vi "5_Manual Window.vi"() -> ()   [LabVIEW 2015]
uses:
  PLC Commucation/Motor cmd setting.ctl
  PLC Commucation/Motor Action.ctl
  PLC Commucation/Motor Selection.ctl
  Variable/Default Setting.ctl
  Variable/Global.vi
  <vilib>/Utility/file.llb/Write To Spreadsheet File (DBL).vi
  <vilib>/Utility/file.llb/Read From Spreadsheet File (DBL).vi
panel:
  in  "Y-Axis-Home":bool
  out "Default Setting":T1
  out "Voltage":dbl
  out "PLC Send CMD":string="*IDN?\n"
  in  "DIGITAL OUTPUT":T2
  in  "Free Axis  RUN":bool
  in  "Free Axis Lock":bool
  in  "Speed(RPM)":i16(knob) max=5000 scale=0.0..5000.0
  in  "X-Axis Save":bool
  in  "Y-Axis Save":bool
  in  "Z-Axis Save":bool
  in  "Z-Axis-Home":bool
  in  "X-Axis-Home":bool
  out "DIGITAL INPUT":T3
  out "Z Actual Position":dbl caption="Actual Position"
  out "Y Actual Position":dbl caption="Actual Position"
  out "X Actual Position":dbl caption="Actual Position"
  in  "Z Axis Run":bool
  in  "Y Axis Run":bool
  in  "X Axis Run":bool
  in  "Z Axis Lock":bool
  in  "X Axis Lock":bool
  in  "Y Axis Lock":bool
  in  "Z-Axis Speed":i16(knob) max=50 scale=0.0..50.0
  in  "Y-Axis Speed":i16(knob) max=50 scale=0.0..50.0
  in  "X-Axis Speed":i16(knob) max=50 scale=0.0..50.0
  out "Receieve CMD":string
  in  "Motor Setting":T4
  out "exit":bool
  in  "Status":bool[](array[boolean])
  in  "zero":bool
  in  "back":bool
  in  "save":bool
  # "Manual Mode Screen"
  # "FREE-Axis"
  # "X-Axis"
  # "Y-Axis"
  # "Z-Axis"
  # "Developed by: VR Engineers"
  # "Contact: 9891971134"
  # "DIGITAL OUTPUT"
  # "DIGITAL OUTPUT"
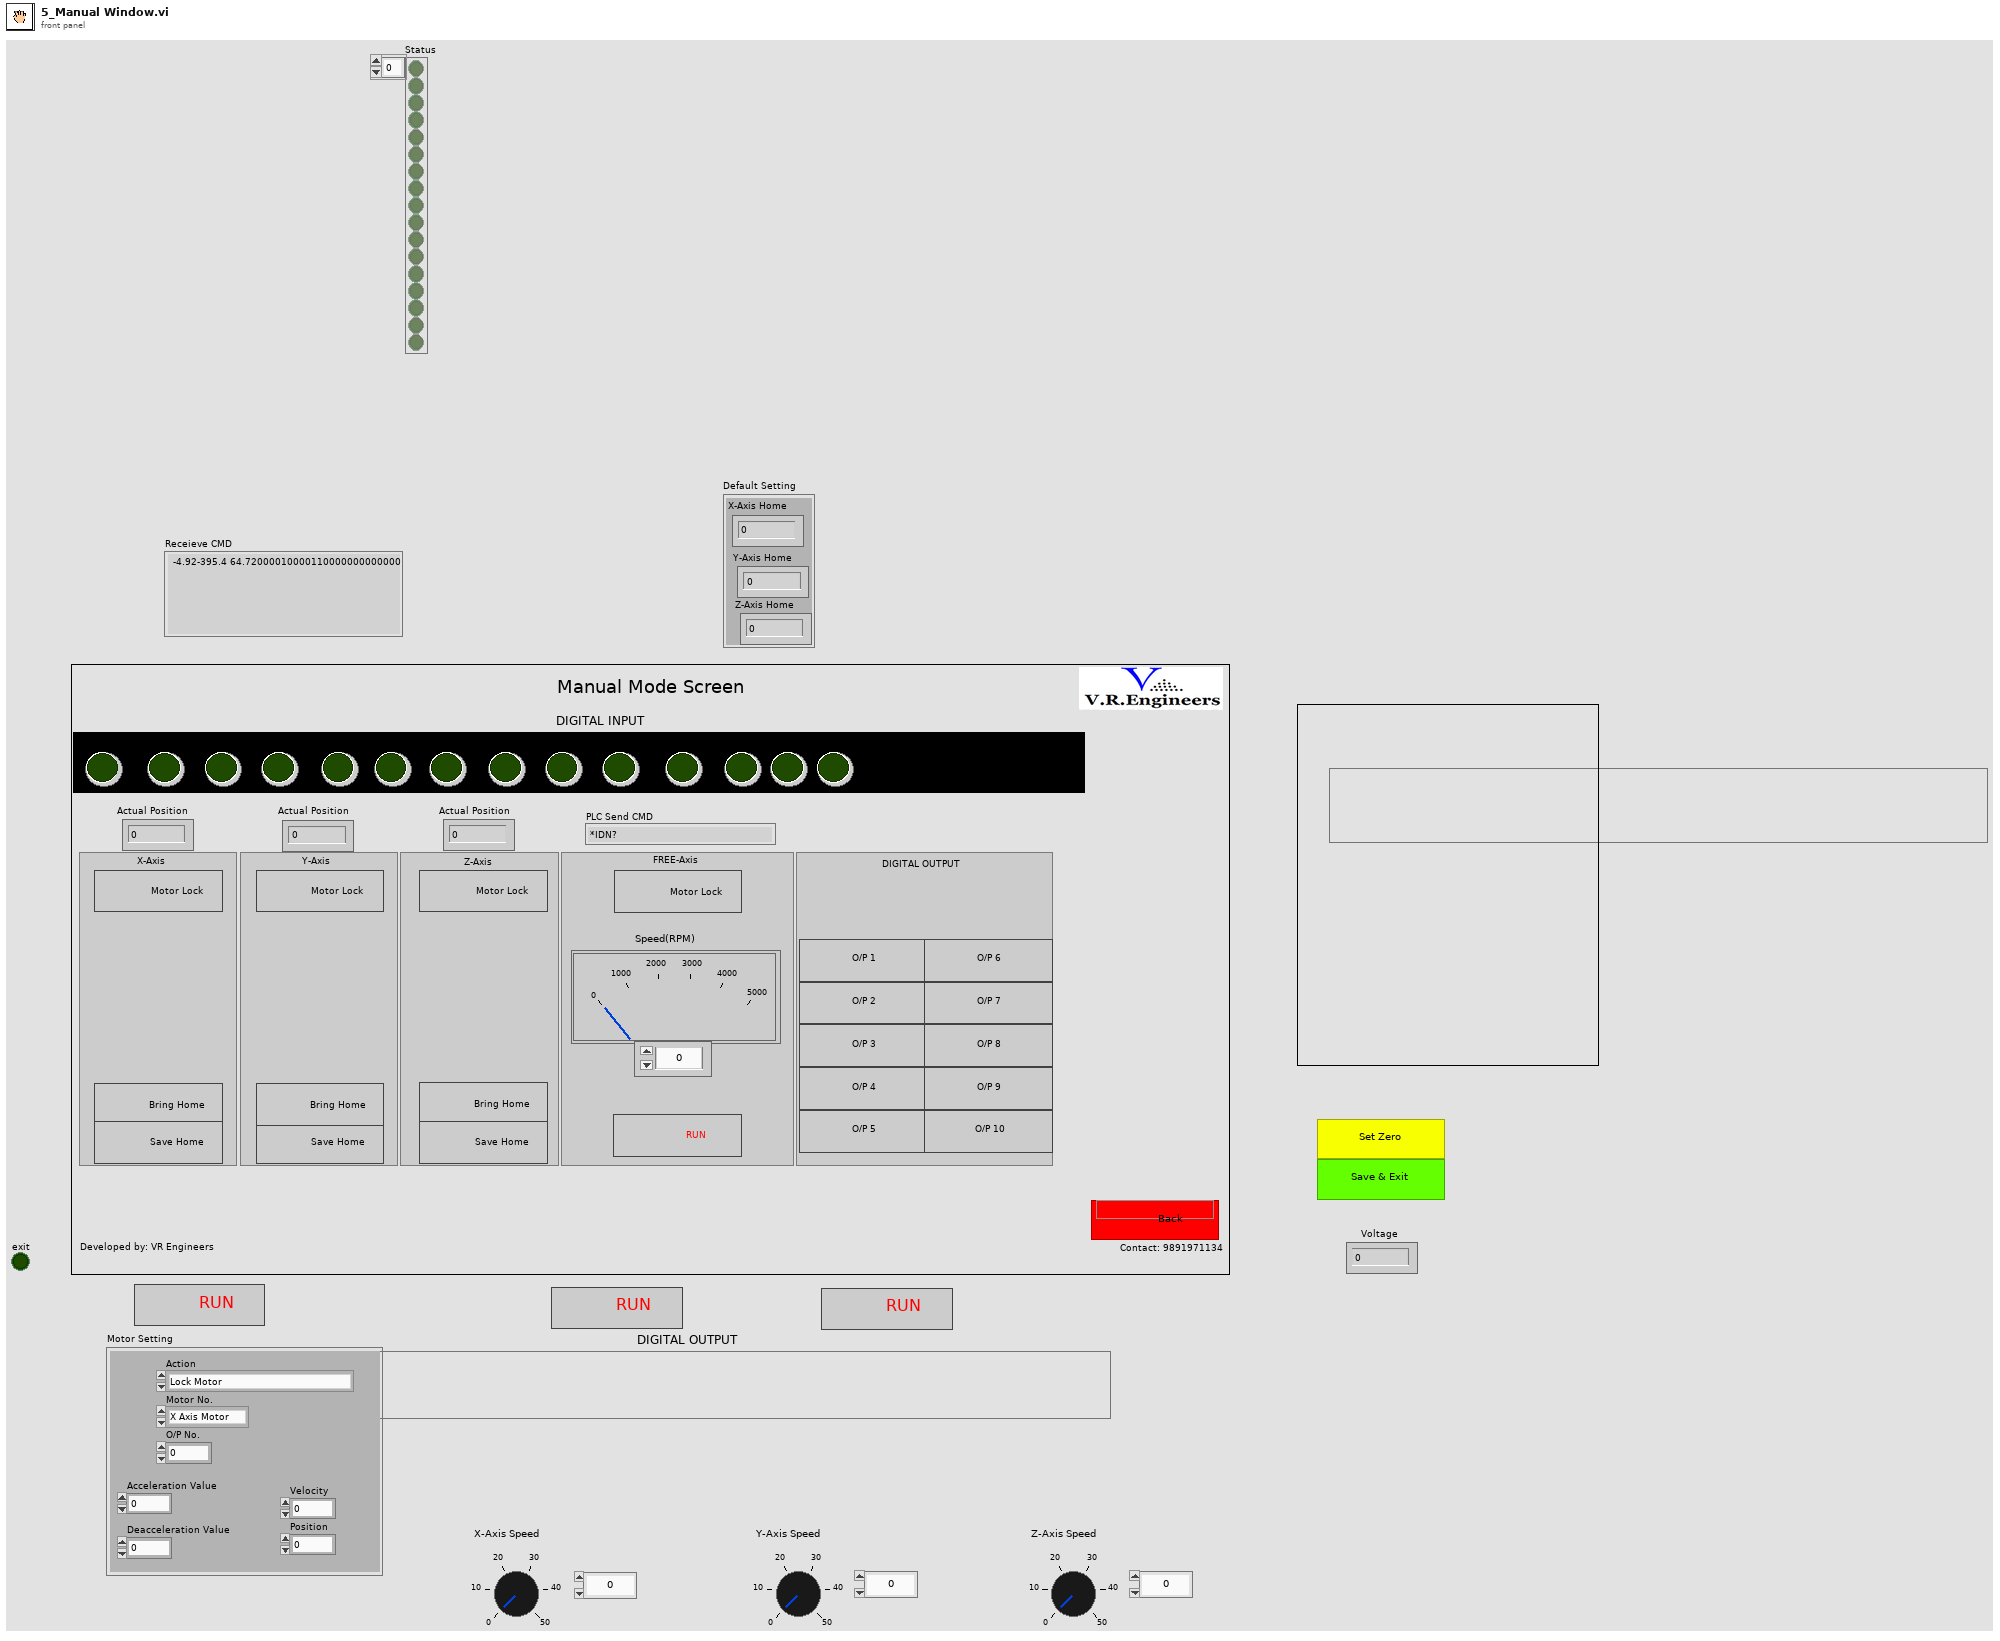
[diagram p1: front panel]
types:
  T1 = typedef "Default Setting.ctl" = cluster{"X-Axis Home":dbl, "Y-Axis Home":dbl, "Z-Axis Home":dbl}
  T2 = cluster{"0":bool, "1":bool, "2":bool, "3":bool, "4":bool, "5":bool, "6":bool, "7":bool, "8":bool, "9":bool}
  T3 = cluster{"Y Axis FWD":bool, "Z Axis DOWN":bool, "Z Axis UP":bool, "X Axis RIGHT":bool, "Y Axis REV":bool, "X Axis LEFT":bool, "X Axis Start":bool, "Y Axis Start":bool, "Z Axis Start":bool, "Emergency":bool, "JOG FWD/REV":bool, "SPI_0011":bool, "SPI_0012":bool, "SPI_0013":bool}
  T4 = typedef "Motor cmd setting.ctl" = cluster{"Action":T5, "Motor No.":T6, "O/P No.":i16, "Acceleration Value":dbl, "Deacceleration Value":dbl, "Position":dbl, "Velocity":dbl}
  T5 = typedef "Motor Action.ctl" = enum16{"Lock Motor", "Unlock Motor", "Set Position Value", "Set Velocity", "Set Acceleration", "Set Deceleration", "Start Motor", "Stop Motor", "Set Home Position", "ALL Servo Home", "Output ON", "Outout OFF"}
  T6 = typedef "Motor Selection.ctl" = enum16{"X Axis Motor", "Y Axis Motor", "Z Axis Motor", "Free Axis Motor"}
  T7 = enum16{"open", "replace", "create", "open or create", "replace or create", "replace or create with confirmation"}
  T8 = enum16{"big-endian, network order", "native, host order", "little-endian"}
  T9 = cluster{"DI[0]":bool, "DI[1]":bool, "DI[2]":bool, "DI[3]":bool, "DI[4]":bool, "DI[5]":bool, "DI[6]":bool, "DI[7]":bool, "DI[8]":bool, "DI[9]":bool, "DI[10]":bool, "DI[11]":bool, "DI[12]":bool, "DI[13]":bool}
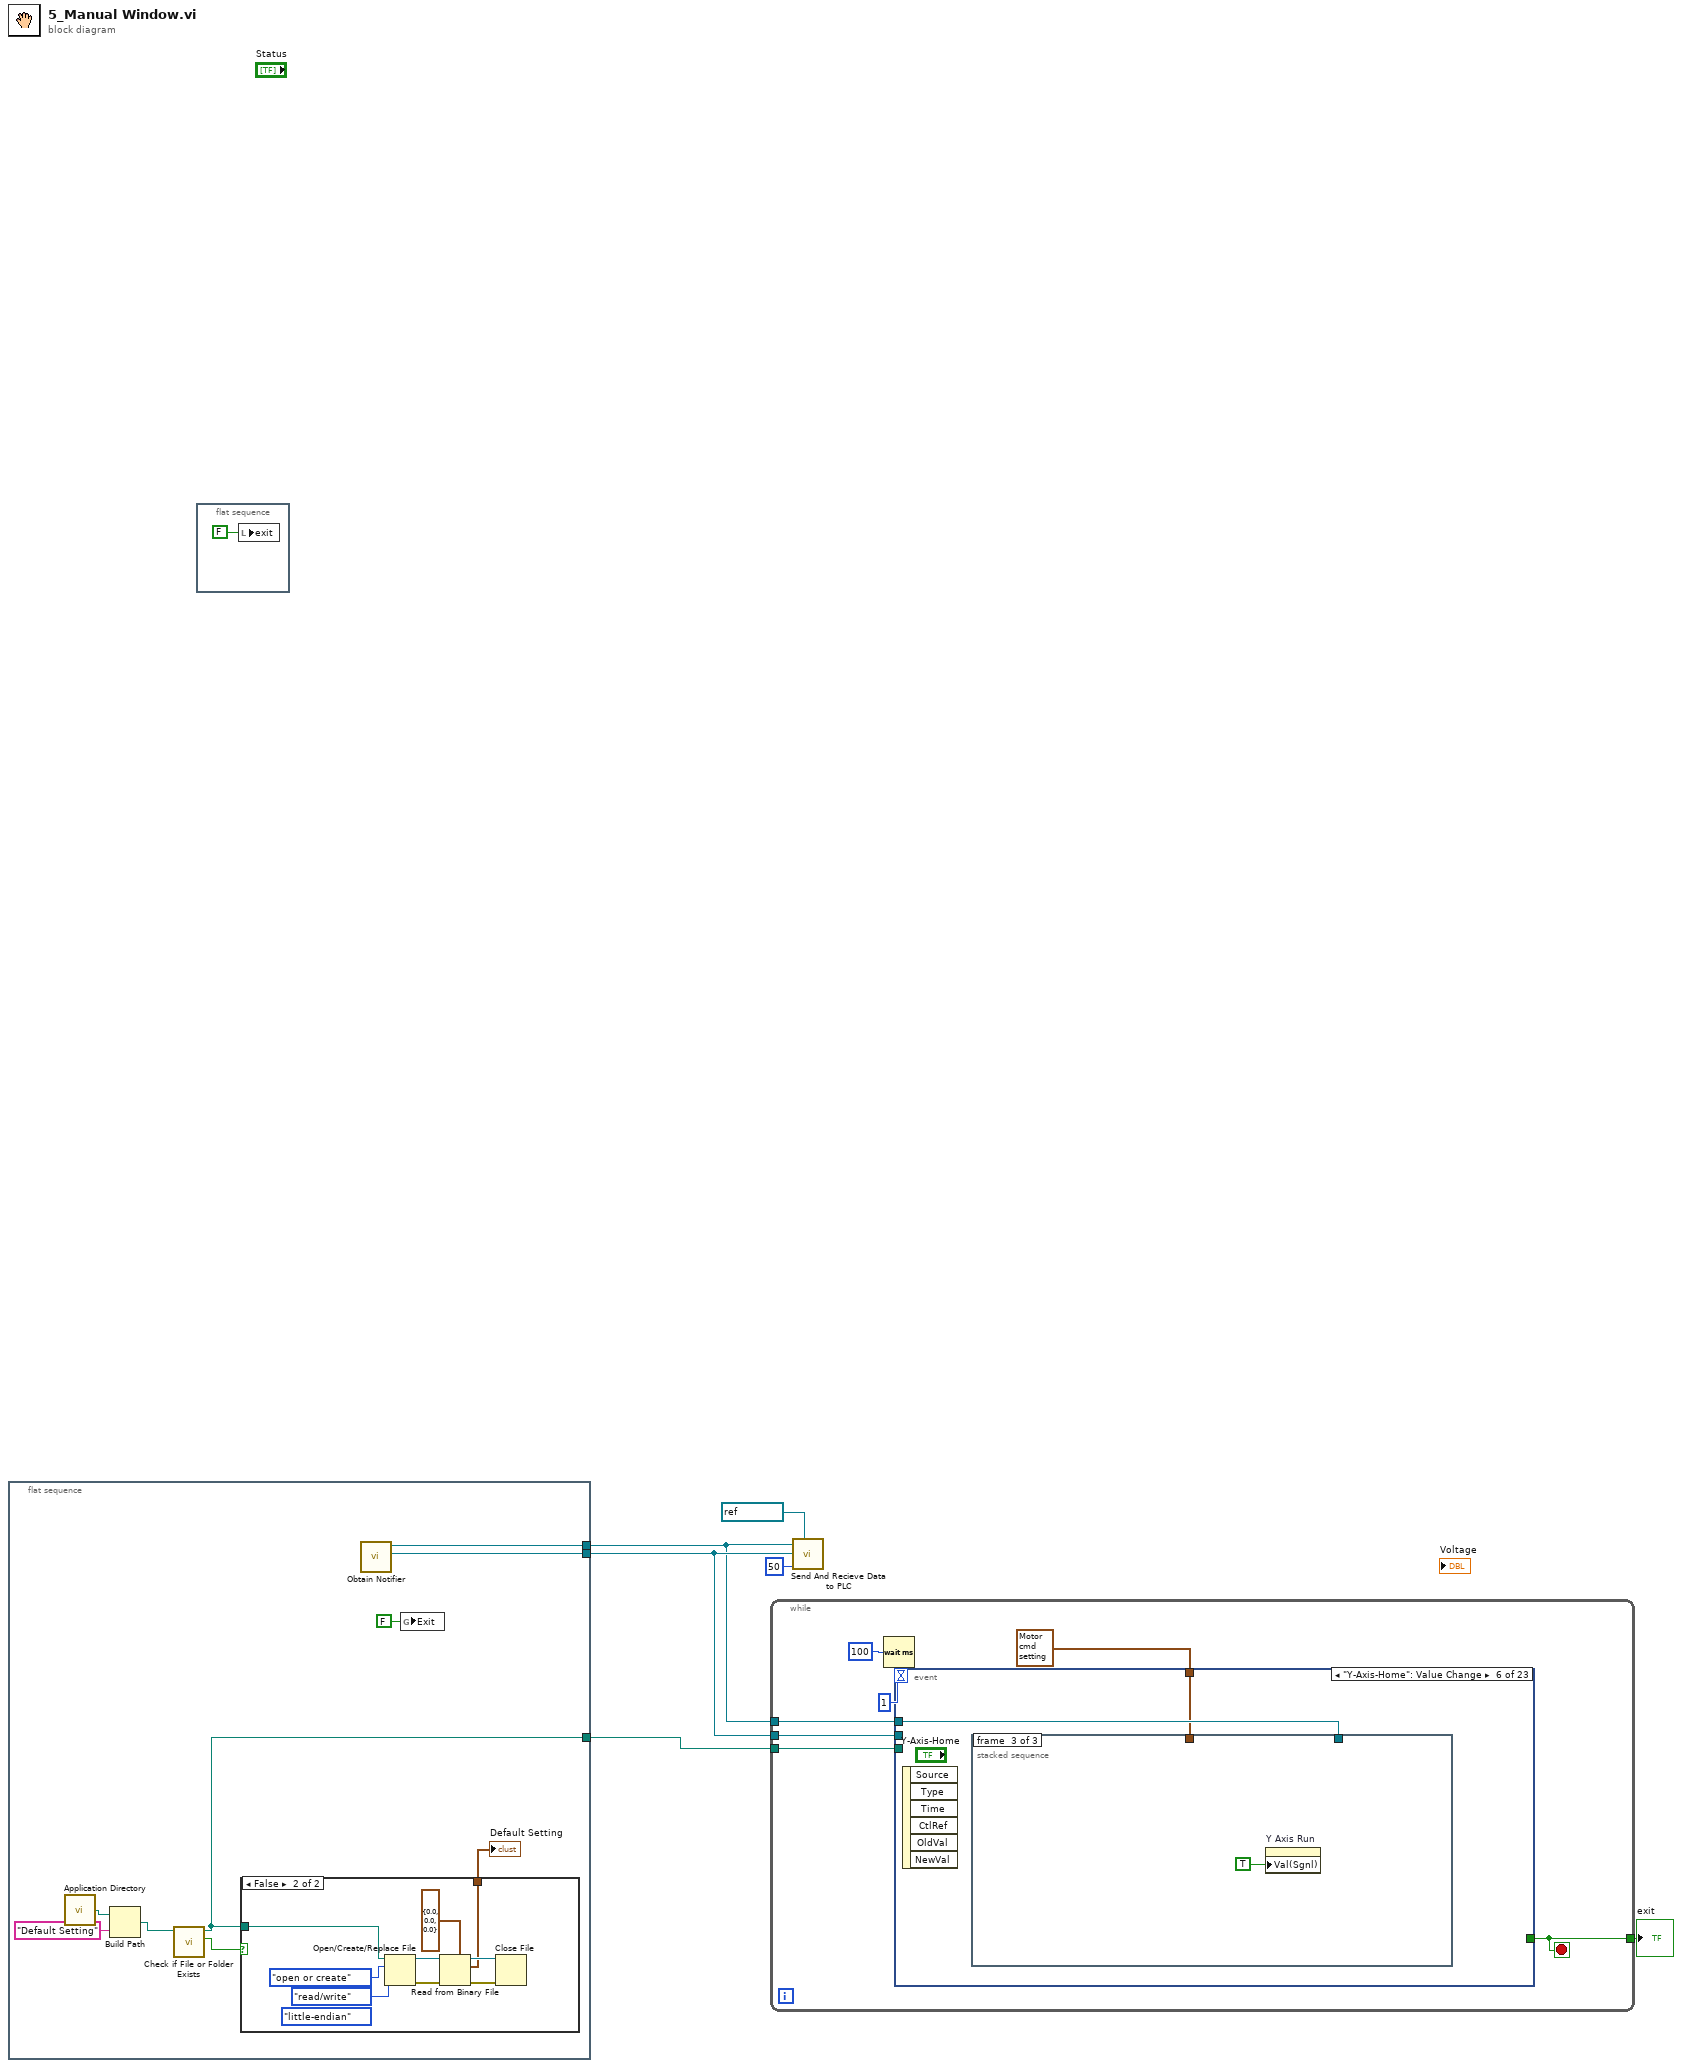
[diagram p0: block diagram]
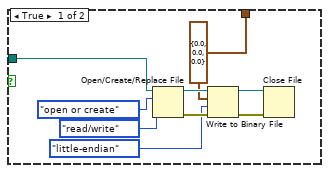
[diagram p2: hidden frame]
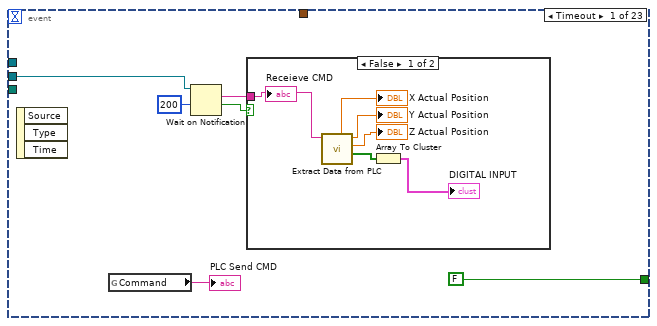
[diagram p3: hidden frame]
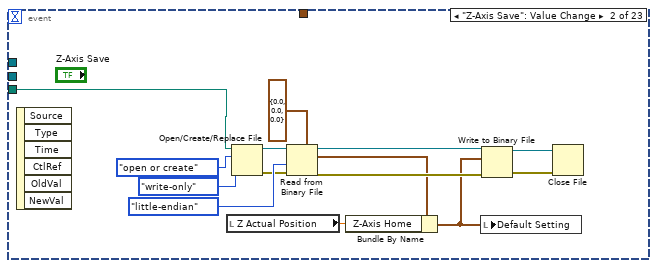
[diagram p5: hidden frame]
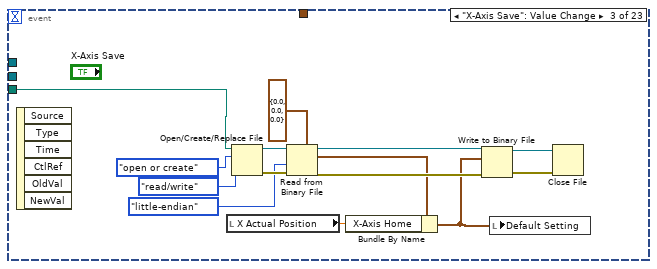
[diagram p6: hidden frame]
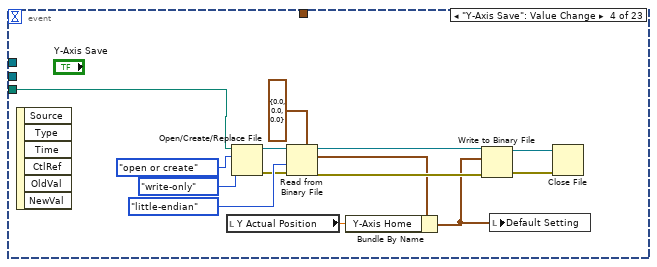
[diagram p7: hidden frame]
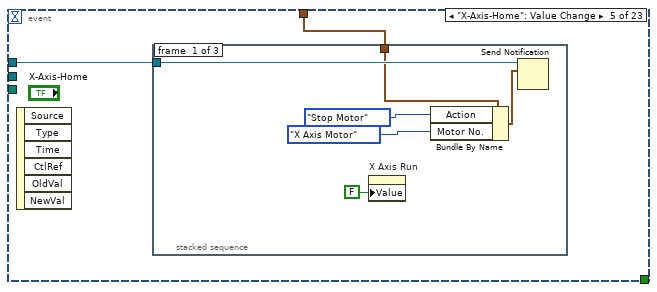
[diagram p8: hidden frame]
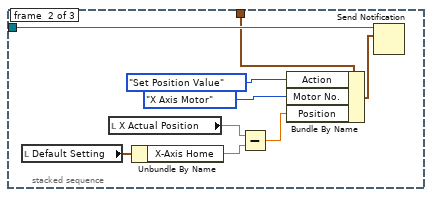
[diagram p9: hidden frame]
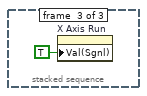
[diagram p10: hidden frame]
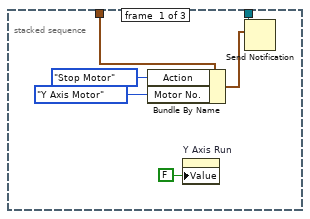
[diagram p11: hidden frame]
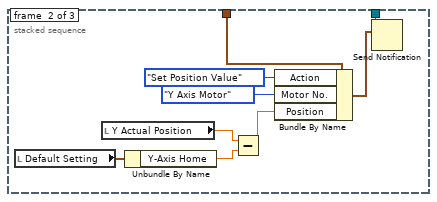
[diagram p12: hidden frame]
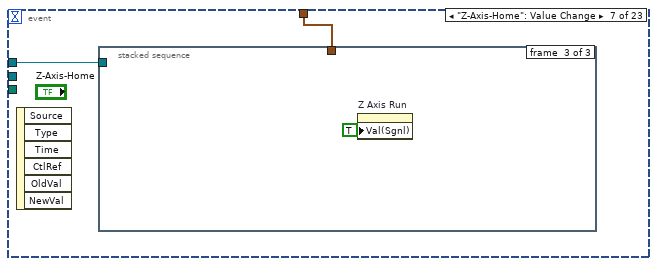
[diagram p13: hidden frame]
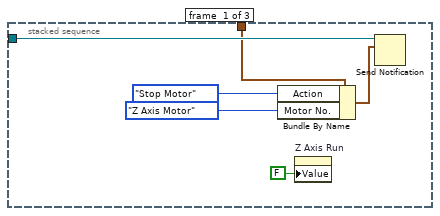
[diagram p14: hidden frame]
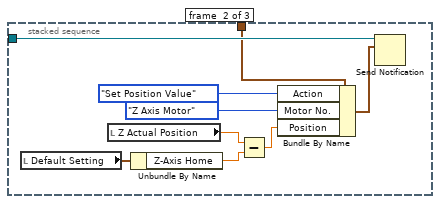
[diagram p15: hidden frame]
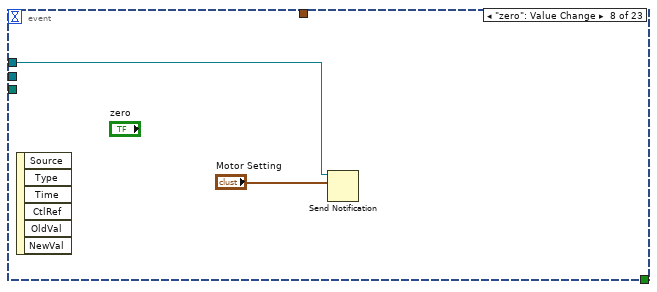
[diagram p16: hidden frame]
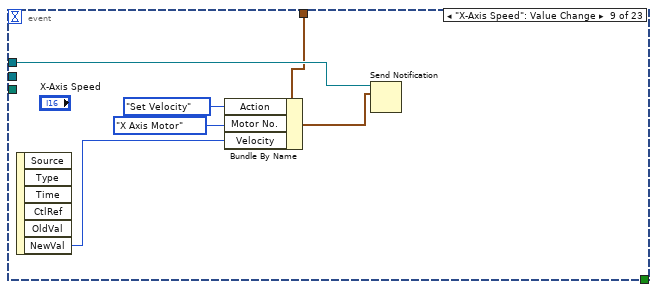
[diagram p17: hidden frame]
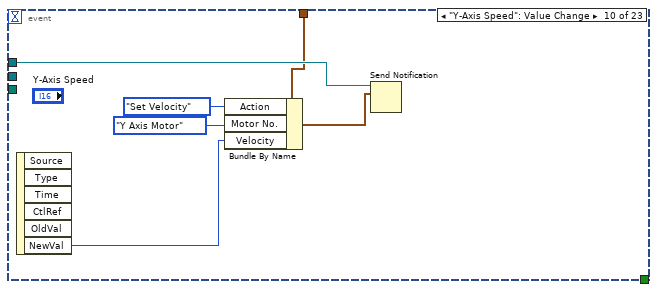
[diagram p18: hidden frame]
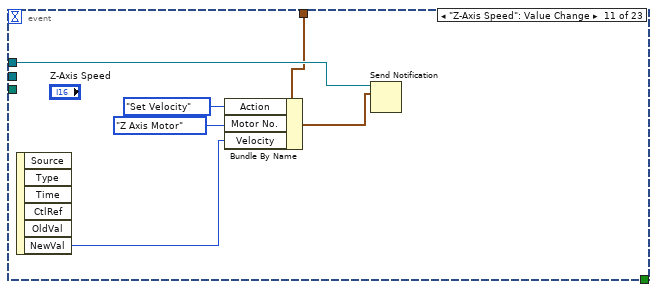
[diagram p19: hidden frame]
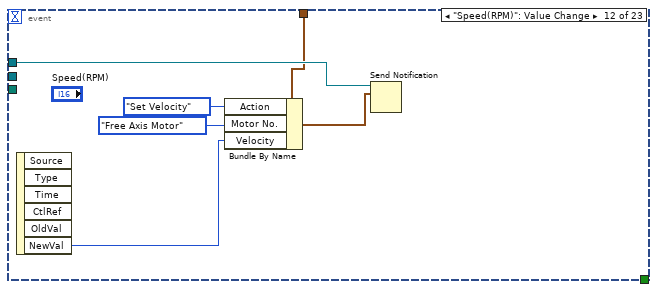
[diagram p20: hidden frame]
diagram:
  n1 = flat-sequence {
    tunnel: [w15] -> w4
    tunnel: [w13] -> w5
    tunnel: [w7] -> w1
    frame #0 {
      n2 = call <vilib>:"Application Directory.vi"() -> ("Application Directory"=w11:path)
      n3 = Build Path(base path=w11, name or relative path="Default Setting") -> (appended path=w8:path)
      n4 = call <vilib>:"Check if File or Folder Exists.vi"("path"=w8) -> ("file or folder exists?"=w9:bool, "dup path"=w7:path)  [unwired: 8 in, 1 out]
      n5 = case shown="False" w9 {
        tunnel: w7 -> [w18 w26]
        tunnel: [w17 w25] -> w10
        frame True {
          w17 = T1 {"X-Axis Home"=0.0, "Y-Axis Home"=0.0, "Z-Axis Home"=0.0} ("Default Setting")
          n6 = Open/Create/Replace File(file path (use dialog)=w18, operation (0:open)=T7."open or create", access (0:read/write)=enum16{"read/write", "read-only", "write-only"}."read/write") -> (refnum out=w20:refnum<file>, error out=w19:errorcluster)  [unwired: 3 in, 1 out]
          n7 = Write to Binary File(file (use dialog)=w20, data=w17, error in=w19, 9:T8."little-endian" ("byte order")) -> (refnum out=w24:refnum<file>, error out=w23:errorcluster)  [unwired: 2 in, 1 out]
          n8 = Close File(refnum=w24, error in=w23) -> ()  [unwired: 2 out]
        }
        frame False {
          (unwired) T8."little-endian" ("byte order")
          n9 = Open/Create/Replace File(file path (use dialog)=w26, operation (0:open)=T7."open or create", access (0:read/write)=enum16{"read/write", "read-only", "write-only"}."read/write") -> (refnum out=w29:refnum<file>, error out=w28:errorcluster)  [unwired: 3 in, 1 out]
          n10 = Read from Binary File(5:T1 {"X-Axis Home"=0.0, "Y-Axis Home"=0.0, "Z-Axis Home"=0.0} ("Default Setting"), 8:w28, 11:w29) -> (0:w32:errorcluster, 2:w25:T1, 3:w33:refnum<file>)  [unwired: 3 in, 1 out]
          n11 = Close File(refnum=w33, error in=w32) -> ()  [unwired: 2 out]
        }
      }
      "Default Setting" <- w10
      n12 = call "Obtain Notifier.vi"() -> ("CMD"=w13:refnum<notifier>, "Setting"=w15:refnum<notifier>)  [unwired: 10 in]
      n13 = global write "Global.vi" "Exit"(FALSE ("Exit")) -> ()
    }
  }
  n14 = flat-sequence {
    frame #0 {
      n15 = local write "exit"(FALSE ("exit")) -> ()
    }
  }
  n16 = while {
    tunnel: [w39] -> w6
    tunnel: w5 -> [w38]
    tunnel: w4 -> [w37]
    tunnel: w1 -> [w35]
    stop <- w39 stop-if-true
    n17 = Wait (ms)(milliseconds to wait=u32 100) -> ()  [unwired: 1 out]
    n18 = event shown="[5] \"Y-Axis-Home\": Value Change" {
      selector: _ -> [_ _ _ _ _ _ _ _ _ _ _ _ _ _ _ _ _ _ _ _ _ _ _]
      dyn-events: _ -> [_ _ _ _ _ _ _ _ _ _ _ _ _ _ _ _ _ _ _ _ _ _ _]
      timeout: 1 -> [_ _ _ _ _ _ _ _ _ _ _ _ _ _ _ _ _ _ _ _ _ _ _]
      tunnel: [FALSE _ _ _ _ _ _ _ _ _ _ _ _ _ _ _ _ _ _ _ _ TRUE TRUE] -> w39
      tunnel: w38 -> [w46 _ _ _ _ _ _ _ _ _ _ _ _ _ _ _ _ _ _ _ _ _ _]
      tunnel: w37 -> [_ _ _ _ w97 w115 w133 w150 w157 w163 w169 w175 w179 w191 w203 w215 w227 w239 w251 w263 w279 _ _]
      tunnel: T4 {"Action"=enum."Lock Motor", "Motor No."=enum."X Axis Motor", "O/P No."=0, "Acceleration Value"=0.0, "Deacceleration Value"=0.0, "Position"=0.0, "Velocity"=0.0} ("Motor Setting") -> [_ _ _ _ w96 w114 w132 _ w156 w162 w168 w174 w178 w190 w202 w214 w226 w238 w250 w262 w278 _ _]
      tunnel: w35 -> [_ w61 w76 w89 _ _ _ _ _ _ _ _ _ _ _ _ _ _ _ _ _ _ _]
      event Timeout {
        n19 = event-data() -> ()  [unwired: 1 in, 3 out]
        n20 = global read "Global.vi" "Command"() -> (→"PLC Send CMD":string)
        n21 = Wait on Notification(notifier=w46, timeout in ms (-1)=200) -> (notification=w44:string, timed out?=w43:bool)  [unwired: 2 in, 2 out]
        n22 = case shown="False" w43 {
          tunnel: w44 -> [w53 _]
          frame False {
            n23 = call "Extract Data from PLC.vi"("Receieve CMD"=w53) -> ("DI"=w49:bool[], "Z Axis Motor"=→"Z Actual Position":dbl, "Y Axis Motor"=→"Y Actual Position":dbl, "X Axis Motor"=→"X Actual Position":dbl)  [unwired: 6 in, 1 out]
            n24 = Array To Cluster(array=w49) -> (cluster=→"DIGITAL INPUT":T9)
            "Receieve CMD" <- w53
          }
          frame True {
          }
        }
      }
      event "Z-Axis Save": Value Change {
        n25 = event-data() -> ()  [unwired: 1 in, 6 out]
        n26 = local read "Z Actual Position"() -> (w55:dbl)
        n27 = Open/Create/Replace File(file path (use dialog)=w61, operation (0:open)=T7."open or create", access (0:read/write)=enum16{"read/write", "read-only", "write-only"}."write-only") -> (refnum out=w64:refnum<file>, error out=w63:errorcluster)  [unwired: 3 in, 1 out]
        n28 = Read from Binary File(5:T1 {"X-Axis Home"=0.0, "Y-Axis Home"=0.0, "Z-Axis Home"=0.0} ("Default Setting"), 8:w63, 9:T8."little-endian" ("byte order"), 11:w64) -> (0:w59:errorcluster, 2:w56:T1, 3:w60:refnum<file>)  [unwired: 2 in, 1 out]
        n29 = Bundle By Name(cluster=w56, "Z-Axis Home"=w55) -> (w54:T1)
        n30 = local write "Default Setting"(w54) -> ()
        n31 = Write to Binary File(file (use dialog)=w60, data=w54, error in=w59) -> (refnum out=w58:refnum<file>, error out=w57:errorcluster)  [unwired: 3 in, 1 out]
        n32 = Close File(refnum=w58, error in=w57) -> ()  [unwired: 2 out]
      }
      event "X-Axis Save": Value Change {
        n33 = event-data() -> ()  [unwired: 1 in, 6 out]
        n34 = local read "X Actual Position"() -> (w70:dbl)
        n35 = Open/Create/Replace File(file path (use dialog)=w76, operation (0:open)=T7."open or create", access (0:read/write)=enum16{"read/write", "read-only", "write-only"}."read/write") -> (refnum out=w79:refnum<file>, error out=w78:errorcluster)  [unwired: 3 in, 1 out]
        n36 = Read from Binary File(5:T1 {"X-Axis Home"=0.0, "Y-Axis Home"=0.0, "Z-Axis Home"=0.0} ("Default Setting"), 8:w78, 9:T8."little-endian" ("byte order"), 11:w79) -> (0:w74:errorcluster, 2:w71:T1, 3:w75:refnum<file>)  [unwired: 2 in, 1 out]
        n37 = Bundle By Name(cluster=w71, "X-Axis Home"=w70) -> (w69:T1)
        n38 = Write to Binary File(file (use dialog)=w75, data=w69, error in=w74) -> (refnum out=w73:refnum<file>, error out=w72:errorcluster)  [unwired: 3 in, 1 out]
        n39 = local write "Default Setting"(w69) -> ()
        n40 = Close File(refnum=w73, error in=w72) -> ()  [unwired: 2 out]
      }
      event "Y-Axis Save": Value Change {
        n41 = event-data() -> ()  [unwired: 1 in, 6 out]
        n42 = local read "Y Actual Position"() -> (w83:dbl)
        n43 = Open/Create/Replace File(file path (use dialog)=w89, operation (0:open)=T7."open or create", access (0:read/write)=enum16{"read/write", "read-only", "write-only"}."write-only") -> (refnum out=w92:refnum<file>, error out=w91:errorcluster)  [unwired: 3 in, 1 out]
        n44 = Read from Binary File(5:T1 {"X-Axis Home"=0.0, "Y-Axis Home"=0.0, "Z-Axis Home"=0.0} ("Default Setting"), 8:w91, 9:T8."little-endian" ("byte order"), 11:w92) -> (0:w87:errorcluster, 2:w84:T1, 3:w88:refnum<file>)  [unwired: 2 in, 1 out]
        n45 = Bundle By Name(cluster=w84, "Y-Axis Home"=w83) -> (w82:T1)
        n46 = Write to Binary File(file (use dialog)=w88, data=w82, error in=w87) -> (refnum out=w86:refnum<file>, error out=w85:errorcluster)  [unwired: 3 in, 1 out]
        n47 = local write "Default Setting"(w82) -> ()
        n48 = Close File(refnum=w86, error in=w85) -> ()  [unwired: 2 out]
      }
      event "X-Axis-Home": Value Change {
        n49 = event-data() -> ()  [unwired: 1 in, 6 out]
        n50 = stacked-sequence {
          tunnel: w97 -> [w103 w110 _]
          tunnel: w96 -> [w102 w109 _]
          frame #0 {
            n51 = property on="X Axis Run" class="Bool (strict)"("Value"=FALSE ("Value (Signaling)")) -> ()  [unwired: 2 in, 2 out]
            n52 = Bundle By Name(cluster=w102, "Action"=Motor_Action."Stop Motor", "Motor No."=Motor_Selection."X Axis Motor") -> (w99:T4)
            n53 = Send Notification(notification=w99, notifier=w103) -> ()  [unwired: 1 in, 2 out]
          }
          frame #1 {
            n54 = local read "Default Setting"() -> (w112:T1)
            n55 = local read "X Actual Position"() -> (w105:dbl)
            n56 = Unbundle By Name(w112) -> ("X-Axis Home"=w111:dbl)
            n57 = Subtract(x=w105, y=w111) -> (x-y=w104:dbl)
            n58 = Bundle By Name(cluster=w109, "Action"=Motor_Action."Set Position Value", "Motor No."=Motor_Selection."X Axis Motor", "Position"=w104) -> (w106:T4)
            n59 = Send Notification(notification=w106, notifier=w110) -> ()  [unwired: 1 in, 2 out]
          }
          frame #2 {
            n60 = property on="X Axis Run" class="Bool (strict)"("Val(Sgnl)"=TRUE ("Value (Signaling)")) -> ()  [unwired: 2 in, 2 out]
          }
        }
      }
      event "Y-Axis-Home": Value Change {
        n61 = event-data() -> ()  [unwired: 1 in, 6 out]
        n62 = stacked-sequence {
          tunnel: w115 -> [w121 w127 _]
          tunnel: w114 -> [w120 w126 _]
          frame #0 {
            n63 = Bundle By Name(cluster=w120, "Action"=Motor_Action."Stop Motor", "Motor No."=Motor_Selection."Y Axis Motor") -> (w117:T4)
            n64 = property on="Y Axis Run" class="Bool (strict)"("Value"=FALSE ("Y Axis Run")) -> ()  [unwired: 2 in, 2 out]
            n65 = Send Notification(notification=w117, notifier=w121) -> ()  [unwired: 1 in, 2 out]
          }
          frame #1 {
            n66 = local read "Default Setting"() -> (w130:T1)
            n67 = local read "Y Actual Position"() -> (w128:dbl)
            n68 = Unbundle By Name(w130) -> ("Y-Axis Home"=w129:dbl)
            n69 = Subtract(x=w128, y=w129) -> (x-y=w123:dbl)
            n70 = Bundle By Name(cluster=w126, "Action"=Motor_Action."Set Position Value", "Motor No."=Motor_Selection."Y Axis Motor", "Position"=w123) -> (w122:T4)
            n71 = Send Notification(notification=w122, notifier=w127) -> ()  [unwired: 1 in, 2 out]
          }
          frame #2 {
            n72 = property on="Y Axis Run" class="Bool (strict)"("Val(Sgnl)"=TRUE ("Y Axis Run")) -> ()  [unwired: 2 in, 2 out]
          }
        }
      }
      event "Z-Axis-Home": Value Change {
        n73 = event-data() -> ()  [unwired: 1 in, 6 out]
        n74 = stacked-sequence {
          tunnel: w133 -> [w139 w145 _]
          tunnel: w132 -> [w138 w144 _]
          frame #0 {
            n75 = Bundle By Name(cluster=w138, "Action"=Motor_Action."Stop Motor", "Motor No."=Motor_Selection."Z Axis Motor") -> (w135:T4)
            n76 = property on="Z Axis Run" class="Bool (strict)"("Value"=FALSE ("Z Axis Run")) -> ()  [unwired: 2 in, 2 out]
            n77 = Send Notification(notification=w135, notifier=w139) -> ()  [unwired: 1 in, 2 out]
          }
          frame #1 {
            n78 = local read "Default Setting"() -> (w148:T1)
            n79 = local read "Z Actual Position"() -> (w146:dbl)
            n80 = Unbundle By Name(w148) -> ("Z-Axis Home"=w147:dbl)
            n81 = Subtract(x=w146, y=w147) -> (x-y=w141:dbl)
            n82 = Bundle By Name(cluster=w144, "Action"=Motor_Action."Set Position Value", "Motor No."=Motor_Selection."Z Axis Motor", "Position"=w141) -> (w140:T4)
            n83 = Send Notification(notification=w140, notifier=w145) -> ()  [unwired: 1 in, 2 out]
          }
          frame #2 {
            n84 = property on="Z Axis Run" class="Bool (strict)"("Val(Sgnl)"=TRUE ("Z Axis Run")) -> ()  [unwired: 2 in, 2 out]
          }
        }
      }
      event "zero": Value Change {
        n85 = event-data() -> ()  [unwired: 1 in, 6 out]
        n86 = Send Notification(notification="Motor Setting", notifier=w150) -> ()  [unwired: 1 in, 2 out]
      }
      event "X-Axis Speed": Value Change {
        n87 = event-data() -> ("NewVal"=w152:i16)  [unwired: 1 in, 5 out]
        n88 = Bundle By Name(cluster=w156, "Action"=Motor_Action."Set Velocity", "Motor No."=Motor_Selection."X Axis Motor", "Velocity"=w152) -> (w155:T4)
        n89 = Send Notification(notification=w155, notifier=w157) -> ()  [unwired: 1 in, 2 out]
      }
      event "Y-Axis Speed": Value Change {
        n90 = event-data() -> ("NewVal"=w158:i16)  [unwired: 1 in, 5 out]
        n91 = Bundle By Name(cluster=w162, "Action"=Motor_Action."Set Velocity", "Motor No."=Motor_Selection."Y Axis Motor", "Velocity"=w158) -> (w161:T4)
        n92 = Send Notification(notification=w161, notifier=w163) -> ()  [unwired: 1 in, 2 out]
      }
      event "Z-Axis Speed": Value Change {
        n93 = event-data() -> ("NewVal"=w164:i16)  [unwired: 1 in, 5 out]
        n94 = Bundle By Name(cluster=w168, "Action"=Motor_Action."Set Velocity", "Motor No."=Motor_Selection."Z Axis Motor", "Velocity"=w164) -> (w167:T4)
        n95 = Send Notification(notification=w167, notifier=w169) -> ()  [unwired: 1 in, 2 out]
      }
      event "Speed(RPM)": Value Change {
        n96 = event-data() -> ("NewVal"=w170:i16)  [unwired: 1 in, 5 out]
        n97 = Bundle By Name(cluster=w174, "Action"=Motor_Action."Set Velocity", "Motor No."=Motor_Selection."Free Axis Motor", "Velocity"=w170) -> (w173:T4)
        n98 = Send Notification(notification=w173, notifier=w175) -> ()  [unwired: 1 in, 2 out]
      }
      event "Free Axis  RUN": Value Change {
        n99 = event-data() -> ("NewVal"=w176:bool)  [unwired: 1 in, 5 out]
        n100 = case shown="True" w176 {
          tunnel: w178 -> [w183 w187]
          tunnel: [w182 w186] -> w177
          frame True {
            n101 = Bundle By Name(cluster=w183, "Action"=Motor_Action."Start Motor", "Motor No."=Motor_Selection."Free Axis Motor") -> (w182:T4)
          }
          frame False {
            n102 = Bundle By Name(cluster=w187, "Action"=Motor_Action."Stop Motor", "Motor No."=Motor_Selection."Free Axis Motor") -> (w186:T4)
          }
        }
        n103 = Send Notification(notification=w177, notifier=w179) -> ()  [unwired: 1 in, 2 out]
      }
      event "X Axis Run": Value Change {
        n104 = event-data() -> ("NewVal"=w188:bool)  [unwired: 1 in, 5 out]
        n105 = case shown="True" w188 {
          tunnel: w190 -> [w195 w199]
          tunnel: [w194 w198] -> w189
          frame True {
            n106 = Bundle By Name(cluster=w195, "Action"=Motor_Action."Start Motor", "Motor No."=Motor_Selection."X Axis Motor") -> (w194:T4)
          }
          frame False {
            n107 = Bundle By Name(cluster=w199, "Action"=Motor_Action."Stop Motor", "Motor No."=Motor_Selection."X Axis Motor") -> (w198:T4)
          }
        }
        n108 = Send Notification(notification=w189, notifier=w191) -> ()  [unwired: 1 in, 2 out]
      }
      event "Y Axis Run": Value Change {
        n109 = event-data() -> ("NewVal"=w200:bool)  [unwired: 1 in, 5 out]
        n110 = case shown="False" w200 {
          tunnel: w202 -> [w207 w211]
          tunnel: [w206 w210] -> w201
          frame True {
            n111 = Bundle By Name(cluster=w207, "Action"=Motor_Action."Start Motor", "Motor No."=Motor_Selection."Y Axis Motor") -> (w206:T4)
          }
          frame False {
            n112 = Bundle By Name(cluster=w211, "Action"=Motor_Action."Stop Motor", "Motor No."=Motor_Selection."Y Axis Motor") -> (w210:T4)
          }
        }
        n113 = Send Notification(notification=w201, notifier=w203) -> ()  [unwired: 1 in, 2 out]
      }
      event "Z Axis Run": Value Change {
        n114 = event-data() -> ("NewVal"=w212:bool)  [unwired: 1 in, 5 out]
        n115 = case shown="False" w212 {
          tunnel: w214 -> [w219 w223]
          tunnel: [w218 w222] -> w213
          frame True {
            n116 = Bundle By Name(cluster=w219, "Action"=Motor_Action."Start Motor", "Motor No."=Motor_Selection."Z Axis Motor") -> (w218:T4)
          }
          frame False {
            n117 = Bundle By Name(cluster=w223, "Action"=Motor_Action."Stop Motor", "Motor No."=Motor_Selection."Z Axis Motor") -> (w222:T4)
          }
        }
        n118 = Send Notification(notification=w213, notifier=w215) -> ()  [unwired: 1 in, 2 out]
      }
      event "Y Axis Lock": Value Change {
        n119 = event-data() -> ("NewVal"=w224:bool)  [unwired: 1 in, 5 out]
        n120 = case shown="False" w224 {
          tunnel: w226 -> [w231 w235]
          tunnel: [w230 w234] -> w225
          frame True {
            n121 = Bundle By Name(cluster=w231, "Action"=Motor_Action."Lock Motor", "Motor No."=Motor_Selection."Y Axis Motor") -> (w230:T4)
          }
          frame False {
            n122 = Bundle By Name(cluster=w235, "Action"=Motor_Action."Unlock Motor", "Motor No."=Motor_Selection."Y Axis Motor") -> (w234:T4)
          }
        }
        n123 = Send Notification(notification=w225, notifier=w227) -> ()  [unwired: 1 in, 2 out]
      }
      event "X Axis Lock": Value Change {
        n124 = event-data() -> ("NewVal"=w236:bool)  [unwired: 1 in, 5 out]
        n125 = case shown="True" w236 {
          tunnel: w238 -> [w243 w247]
          tunnel: [w242 w246] -> w237
          frame True {
            n126 = Bundle By Name(cluster=w243, "Action"=Motor_Action."Lock Motor", "Motor No."=Motor_Selection."X Axis Motor") -> (w242:T4)
          }
          frame False {
            n127 = Bundle By Name(cluster=w247, "Action"=Motor_Action."Unlock Motor", "Motor No."=Motor_Selection."X Axis Motor") -> (w246:T4)
          }
        }
        n128 = Send Notification(notification=w237, notifier=w239) -> ()  [unwired: 1 in, 2 out]
      }
      event "Z Axis Lock": Value Change {
        n129 = event-data() -> ("NewVal"=w248:bool)  [unwired: 1 in, 5 out]
        n130 = case shown="False" w248 {
          tunnel: w250 -> [w255 w259]
          tunnel: [w254 w258] -> w249
          frame True {
            n131 = Bundle By Name(cluster=w255, "Action"=Motor_Action."Lock Motor", "Motor No."=Motor_Selection."Z Axis Motor") -> (w254:T4)
          }
          frame False {
            n132 = Bundle By Name(cluster=w259, "Action"=Motor_Action."Unlock Motor", "Motor No."=Motor_Selection."Z Axis Motor") -> (w258:T4)
          }
        }
        n133 = Send Notification(notification=w249, notifier=w251) -> ()  [unwired: 1 in, 2 out]
      }
      event "Free Axis Lock": Value Change {
        n134 = event-data() -> ("NewVal"=w260:bool)  [unwired: 1 in, 5 out]
        n135 = case shown="True" w260 {
          tunnel: w262 -> [w267 w271]
          tunnel: [w266 w270] -> w261
          frame True {
            n136 = Bundle By Name(cluster=w267, "Action"=Motor_Action."Lock Motor", "Motor No."=Motor_Selection."Free Axis Motor") -> (w266:T4)
          }
          frame False {
            n137 = Bundle By Name(cluster=w271, "Action"=Motor_Action."Unlock Motor", "Motor No."=Motor_Selection."Free Axis Motor") -> (w270:T4)
          }
        }
        n138 = Send Notification(notification=w261, notifier=w263) -> ()  [unwired: 1 in, 2 out]
      }
      event "DIGITAL OUTPUT.0", "DIGITAL OUTPUT.1", "DIGITAL OUTPUT.2", "DIGITAL OUTPUT.3", "DIGITAL OUTPUT.4", "DIGITAL OUTPUT.5", "DIGITAL OUTPUT.6", "DIGITAL OUTPUT.7", "DIGITAL OUTPUT.8", "DIGITAL OUTPUT.9": Value Change {
        n139 = event-data() -> ("NewVal"=w282:bool, "CtlRef"=w274:refnum<vi>)  [unwired: 1 in, 5 out]
        n140 = property class="Bool"(reference=w274) -> ("Label.Text"=w281:string)  [unwired: 1 in, 2 out]
        n141 = Fract/Exp String To Number(string=w281, default (0 dbl)=i16 0 ("default (0 DBL)")) -> (number=w273:i16)  [unwired: 2 in, 1 out]
        n142 = Select(t=Motor_Action."Output ON" ("Action"), s=w282, f=Motor_Action."Outout OFF" ("Action")) -> (s? t:f=w275:T5)
        n143 = Bundle By Name(cluster=w278, "Action"=w275, "O/P No."=w273) -> (w272:T4)
        n144 = Send Notification(notification=w272, notifier=w279) -> ()  [unwired: 1 in, 2 out]
      }
      event "save": Value Change {
        n145 = event-data() -> ()  [unwired: 1 in, 6 out]
        n146 = disable-structure shown="Disabled" {
          disable-tunnel: _ -> [w284 _]
          frame Disabled {
            n147 = call-poly <vilib>:"Write To Spreadsheet File.vi"("append to file? (new file:F)"=FALSE, "file path (dialog if empty)"=w284) -> ("new file path (Not A Path if cancelled)"=w292:path, "2D data"=w293:dbl[][])  [unwired: 5 in]
            n148 = call-poly <vilib>:"Read From Spreadsheet File.vi"("file path (dialog if empty)"=w292) -> ("all rows"=w291:dbl[][])  [unwired: 6 in, 4 out]
            n149 = Index Array(array=w291, index (row) #1=0 ("disabled index (col)"), index (row) #2=1 ("index (col)")) -> (element #1=w294:dbl[], element #2=w298:dbl[])  [unwired: 2 in]
            n150 = Index Array(array=w294, index #1=0 ("index"), index #2=1 ("index")) -> (element #2=w287:dbl)  [unwired: 1 out]
            n151 = Index Array(array=w298, index #1=0 ("index"), index #2=1 ("index"), index #3=2 ("index")) -> ()  [unwired: 3 out]
          }
          frame Enabled {
          }
        }
      }
      event "back": Value Change {
        n152 = event-data() -> ()  [unwired: 1 in, 6 out]
      }
    }
  }
  "exit" <- w6
  n153 = call "Send And Recieve Data to PLC.vi"("VISA resource name"=refnum<visa-resource-name> "COM1", "delay before read (ms)"=u32 50, "CMD"=w5, "Setting"=w4) -> ()  [unwired: 8 in]
